vi "Arduino Master Low Level.vi"(0 "Arduino VISA resource index":i32, 1 "Tx msg cluster":T2={"dest"=1, "A/D/C"="A", "R/W"="R", "chan"=1, "val (float)"=0.0}) -> (2 "Value returned":sgl, 3 "Rx checksum ok?":bool, 4 "Tx checksum ok?":bool, 5 "Error":errorcluster)   [LabVIEW 2013]
uses:
  ctls_and_globals/Arduino tx msg cluster.ctl
  ctls_and_globals/Arduino Config & resource typedef.ctl
  ctls_and_globals/Arduino Global.vi
panel:
  out "Arduino VISA config & resource":T1={"VISA resource name"="COM12", "baud rate (bps)"=276000, "timeout (ms)"=5000, "data bits"=8, "parity"=enum."None", "stop bits (10: 1 bit)"=10, "flow control"=0, "termination char (hex)"=10, "Enable Termination Char"=FALSE, "byte count"=12, "Resource locked?"=FALSE} {"termination char (hex)" format="%02x"; "stop bits (10: 1 bit)" items=["1.0"=10, "1.5"=15, "2.0"=20]; "flow control" items=["None", "XON/XOFF", "RTS/CTS", "XON/XOFF & RTS/CTS", "DTR/DSR", "XON/XOFF & DTR/DSR"]}
  out "Bytes returned":u32
  out "Read buffer (hex)":string
  out "Write buffer (hex)":string
  # "PN custom comms protocol rx / tx msg syntax is 12 bytes: \n'@', src., dest., A/D/C, R/W, chan, val, val ,val, val, rxCHK, txCHK"
  # "Only need to input the following:\ndest, A/D/C, R/W, chan, val, val, val, val\nbyte     str       str    byte            float"
  # "PN 15/07/2013"
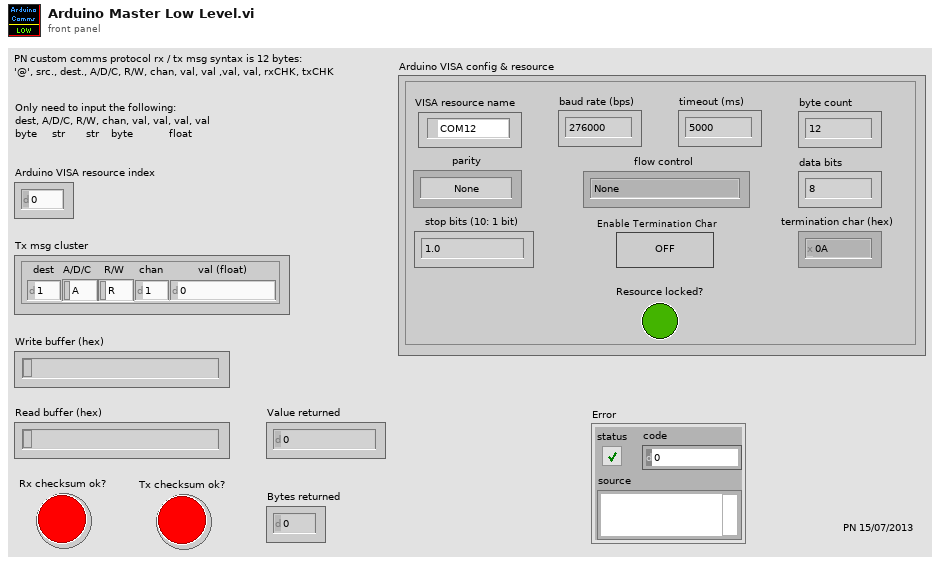
[diagram p1: front panel]
types:
  T1 = typedef "Arduino Config & resource typedef.ctl" = cluster{"VISA resource name":refnum<visa-resource-name>, "baud rate (bps)":u32, "timeout (ms)":u32, "data bits":u16, "parity":enum16{"None", "Odd", "Even", "Mark", "Space"}, "stop bits (10: 1 bit)":u16, "flow control":u16, "termination char (hex)":u8, "Enable Termination Char":bool, "byte count":u32, "Resource locked?":bool}
  T2 = typedef "Arduino tx msg cluster.ctl" = cluster{"dest":u8, "A/D/C":string, "R/W":string, "chan":u8, "val (float)":sgl}
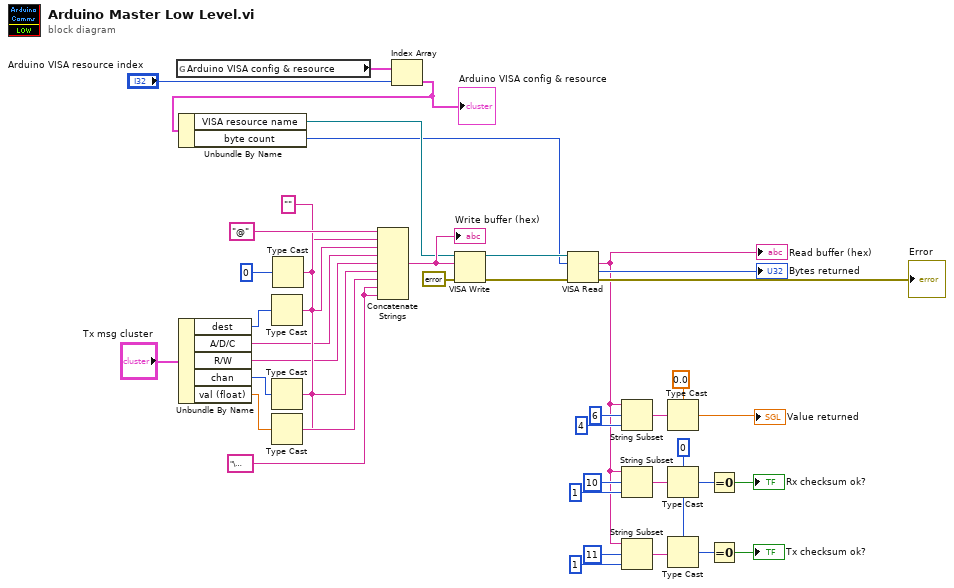
[diagram p0: block diagram]
diagram:
  w23 = u8 0 ("offset (0)")
  w35 = "\u0000"
  w11 = ""
  n1 = global read "Arduino Global.vi" "Arduino VISA config & resource"() -> (w42:T1[])
  n2 = Unbundle By Name("Tx msg cluster") -> ("dest"=w5:u8, "A/D/C"=w4:string, "R/W"=w3:string, "chan"=w2:u8, "val (float)"=w1:sgl)
  n3 = Type Cast(type=w11, x=w5) -> (*(type *) &x=w38:string)
  n4 = Type Cast(type=w11, x=w2) -> (*(type *) &x=w37:string)
  n5 = Type Cast(type=w11, x=w1) -> (*(type *) &x=w36:string)
  n6 = Type Cast(type=w11, x=u8 0) -> (*(type *) &x=w10:string)
  n7 = Concatenate Strings("@", w10, w38, w4, w3, w37, w36, w35, w35) -> (w34:string)
  "Write buffer (hex)" <- w34
  n8 = Index Array(array=w42, index="Arduino VISA resource index") -> (element=w32:T1)
  "Arduino VISA config & resource" <- w32
  n9 = Unbundle By Name(w32) -> ("VISA resource name"=w31:refnum<visa-resource-name>, "byte count"=w26:u32)
  n10 = VISA Write(VISA resource name=w31, write buffer=w34, error in (no error)=errorcluster {"status"=FALSE, "code"=0, "source"=""}) -> (VISA resource name out=w27:refnum<visa-resource-name>, error out=w30:errorcluster)  [unwired: 1 out]
  n11 = VISA Read(VISA resource name=w27, byte count=w26, error in (no error)=w30) -> (read buffer=w14:string, return count=→"Bytes returned":u32, error out=→"Error":errorcluster)  [unwired: 1 out]
  "Read buffer (hex)" <- w14
  n12 = String Subset(string=w14, offset (0)=6, length (rest)=4 ("length (rest)")) -> (substring=w17:string)
  n13 = String Subset(string=w14, offset (0)=10, length (rest)=1 ("length (rest)")) -> (substring=w21:string)
  n14 = String Subset(string=w14, offset (0)=11, length (rest)=1 ("length (rest)")) -> (substring=w22:string)
  n15 = Type Cast(type=sgl 0.0, x=w17) -> (*(type *) &x=→"Value returned":sgl)
  n16 = Type Cast(type=w23, x=w21) -> (*(type *) &x=w24:u8)
  n17 = Type Cast(type=w23, x=w22) -> (*(type *) &x=w25:u8)
  n18 = Equal To 0?(x=w24) -> (x = 0?=→"Rx checksum ok?":bool)
  n19 = Equal To 0?(x=w25) -> (x = 0?=→"Tx checksum ok?":bool)
